vi "7.2 Loop with Shift Registers.vi"() -> ()   [LabVIEW 2019]
panel:
  in  "Stop":bool
  out "Final Result":dbl
  out "Result inside":dbl
  out "Multiply":i32
  out "Sum":i32
  out "2nd total":i32
  out "1st total":i32
  # "OUT OF THE LOOP 1"
  # "INSIDE THE LOOP 1"
  # "LOOP 2"
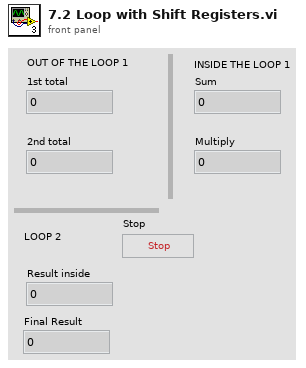
[diagram p1: front panel]
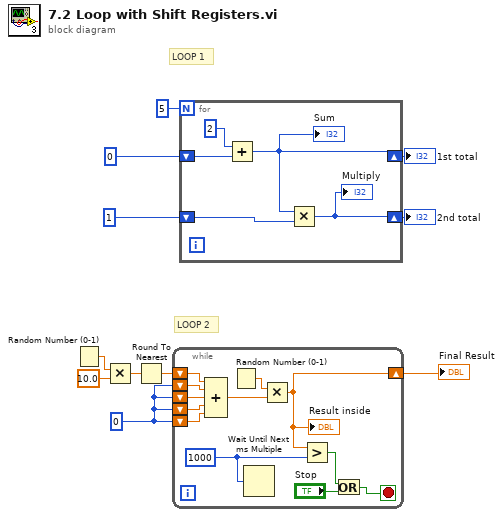
[diagram p0: block diagram]
diagram:
  w1 = 0
  # "LOOP 1"
  # "LOOP 2"
  n1 = Random Number (0-1)() -> (number: 0 to 1=w5:dbl)
  n2 = Multiply(x=w5, y=10.0) -> (x*y=w4:dbl)
  n3 = Round To Nearest(number=w4) -> (nearest integer value=w3:dbl)
  n4 = while {
    shift-right: [w13] -> w2
    shift-left: w3 -> [w23]
    shift-left: w1 -> [w22]
    shift-left: w1 -> [w21]
    shift-left: w1 -> [w20]
    shift-left: w1 -> [w19]
    stop <- w15 stop-if-true
    w12 = u32 1000 ("millisecond multiple")
    n5 = Compound Arithmetic op=ADD(w23, w22, w21, w20, w19) -> (w18:dbl)
    n6 = Random Number (0-1)() -> (number: 0 to 1=w17:dbl)
    n7 = Wait Until Next ms Multiple(millisecond multiple=w12) -> ()  [unwired: 1 out]
    n8 = Multiply(x=w17, y=w18) -> (x*y=w13:dbl)
    "Result inside" <- w13
    n9 = Greater?(x=w13, y=w12) -> (0:w14:bool)
    n10 = Or(x=w14, y="Stop") -> (x .or. y?=w15:bool)
  }
  "Final Result" <- w2
  n11 = for {
    N: 5 -> [_]
    shift-right: [w24] -> w7
    shift-left: 1 -> [w26]
    shift-right: [w25] -> w8
    shift-left: 0 -> [w27]
    n12 = Add(x=2, y=w27) -> (x+y=w25:i32)
    "Sum" <- w25
    n13 = Multiply(x=w25, y=w26) -> (x*y=w24:i32)
    "Multiply" <- w24
  }
  "1st total" <- w8
  "2nd total" <- w7
